vi "Start Channel Stream.vi"(6 "Channel index":i32, 8 "error in (no error)":errorcluster, 9 "Waveform":waveform(i16), 11 "Red Pitaya Digitizer in":refnum<class "Red Pitaya Digitizer.lvclass">) -> (0 "error out":errorcluster, 1 "channel name(s) out":string, 2 "group name out":string, 3 "Red Pitaya Digitizer out":refnum<class "Red Pitaya Digitizer.lvclass">)   [LabVIEW 2016, in "Red Pitaya Digitizer.lvclass"]
uses:
  Red Pitaya Digitizer.lvclass
  C:/github/NHMFL_Core/Libraries/Instruments/Pulse Driver/Pulse Driver.lvclass
  Red Pitaya Digitizer.lvclass/Red Pitaya Digitizer.ctl
  Instruments/Pulse Driver/Pulse Driver.lvclass/Pulse Driver.ctl
  Instruments/Pulse Driver/Read tdms file.vi
  Instruments/Pulse Driver/Write tdms file.vi
  Instruments/Pulse Driver/Pulse Driver.lvclass
  RP Core/RP Instrument/RP Instrument.lvclass
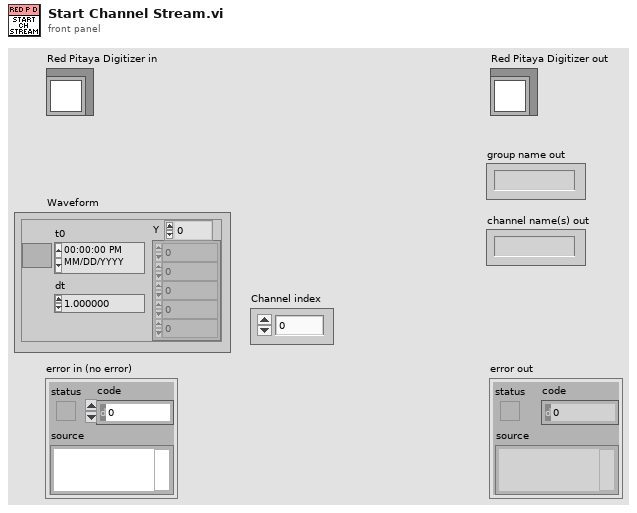
[diagram p1: front panel]
types:
  T1 = typedef "Lockin Parameters.ctl" = cluster{"Frequency":dbl, "Phase":dbl, "Syncronous":bool, "Points per sine wave":i32, "DDS":bool, "Frequency word":u32, "Phase word":u32, "DDS modulus":i64, "DDS clock":dbl}
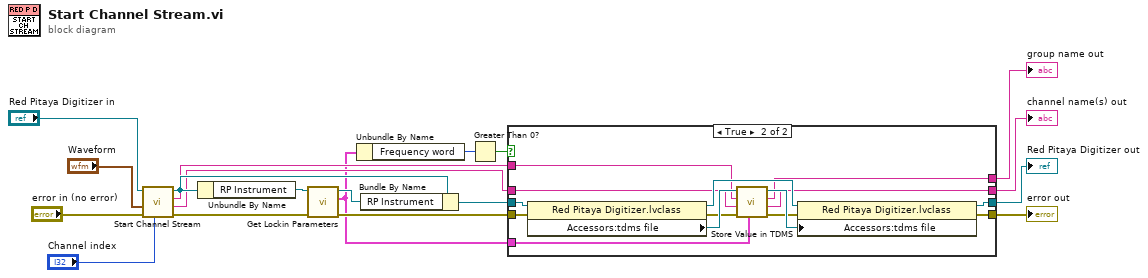
[diagram p0: block diagram]
diagram:
  n1 = call-parent "Start Channel Stream.vi"("Channel index"="Channel index", "error in (no error)"="error in (no error)", "Waveform"="Waveform", "Pulse Driver in"="Red Pitaya Digitizer in") -> ("error out"=w13:errorcluster, "channel name(s) out"=w7:string, "group name out"=w6:string, "Pulse Driver out"=w12:refnum<class "Red Pitaya Digitizer.lvclass">)  [unwired: 4 in]
  n2 = Unbundle By Name(w12) -> ("RP Instrument"=w14:refnum<class "RP Instrument.lvclass">)
  n3 = call-dynamic "Get Lockin Parameters.vi"("error in (no error)"=w13, "RP Instrument in"=w14) -> ("error out"=w8:errorcluster, "Lockin parameters"=w1:T1, "RP Instrument out"=w11:refnum<class "RP Instrument.lvclass">)  [unwired: 7 in]
  n4 = Unbundle By Name(w1) -> ("Frequency word"=w15:u32)
  n5 = Bundle By Name(cluster=w12, "RP Instrument"=w11) -> (w9:refnum<class "Red Pitaya Digitizer.lvclass">)
  n6 = Greater Than 0?(x=w15) -> (x > 0?=w10:bool)
  n7 = case shown="True" w10 {
    tunnel: w9 -> [w21 w37]
    tunnel: w8 -> [w20 w35]
    tunnel: w7 -> [w22 w30]
    tunnel: w6 -> [w23 w29]
    tunnel: [w23 w28] -> w5
    tunnel: [w22 w27] -> w4
    tunnel: [w21 w26] -> w3
    tunnel: [w20 w25] -> w2
    tunnel: w1 -> [_ w24]
    frame False {
    }
    frame True {
      n8 = property class="Red Pitaya Digitizer.lvclass"(reference=w37, error in=w35) -> (reference out=w36:refnum<class "Red Pitaya Digitizer.lvclass">, error out=w32:errorcluster, "Accessors:tdms file"=w34:refnum<k34>)
      n9 = call "Store Value in TDMS.vi"("Value"=w24, "Error In"=w32, "channel name"=w30, "group name"=w29, "tdms file"=w34) -> ("Error Out"=w31:errorcluster, "channel name out"=w27:string, "group name out"=w28:string, "tdms file out"=w33:refnum<k34>)  [unwired: 3 in]
      n10 = property class="Red Pitaya Digitizer.lvclass"(reference=w36, error in=w31, "Accessors:tdms file"=w33) -> (reference out=w26:refnum<class "Red Pitaya Digitizer.lvclass">, error out=w25:errorcluster)
    }
  }
  "error out" <- w2
  "Red Pitaya Digitizer out" <- w3
  "channel name(s) out" <- w4
  "group name out" <- w5
